vi "Refnum_to_data.vi"(8 "error in (no error)":errorcluster, 11 "refnum in":T1) -> (0 "error out":errorcluster, 3 "DAQ refnum out":refnum<visa-resource-name>, 4 "delay out":u32)   [LabVIEW 2018, in "Korad KA3305P.lvlib"]
uses:
  Korad KA3305P.lvlib
  Reference.ctl
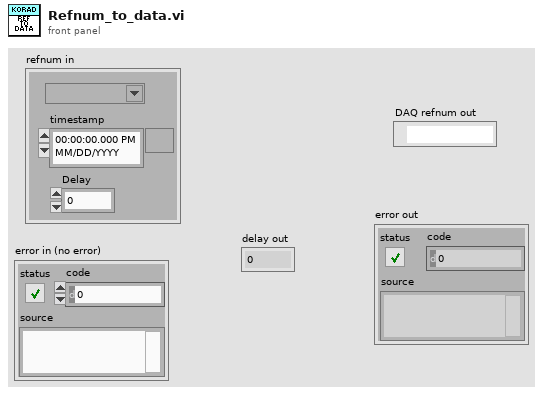
[diagram p1: front panel]
types:
  T1 = typedef "Korad KA3305P.lvlib/Reference.ctl" = cluster{"refnum":refnum<visa-resource-name>, "timestamp":timestamp, "Delay":dbl}
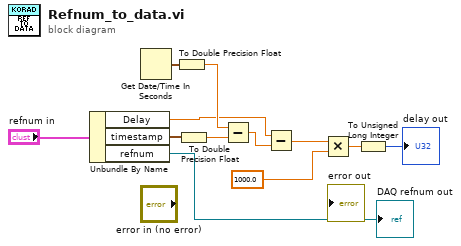
[diagram p0: block diagram]
diagram:
  n1 = Unbundle By Name("refnum in") -> ("Delay"=w3:dbl, "timestamp"=w8:timestamp, "refnum"=→"DAQ refnum out":refnum<visa-resource-name>)
  n2 = Get Date/Time In Seconds() -> (seconds since 1Jan1904=w9:timestamp)
  n3 = To Double Precision Float(number=w9) -> (double precision float=w6:dbl)
  n4 = To Double Precision Float(number=w8) -> (double precision float=w7:dbl)
  n5 = Subtract(x=w6, y=w7) -> (x-y=w5:dbl)
  n6 = Subtract(x=w3, y=w5) -> (x-y=w12:dbl)
  n7 = Multiply(x=w12, y=1000.0) -> (x*y=w10:dbl)
  n8 = To Unsigned Long Integer(number=w10) -> (unsigned 32bit integer=→"delay out":u32)
